vi "Ctor.vi"(8 "error in (no error)":errorcluster, 11 "SinglePlotPanel (type)":refnum<class "RocketPlotPanel.lvclass">) -> (0 "error out":errorcluster, 3 "SinglePlotPanel (running type)":refnum<class "RocketPlotPanel.lvclass">)   [LabVIEW 2021, in "RocketPlot.lvlib" / "RocketPlotPanel.lvclass"]
uses:
  RocketPlotPanel.lvclass
  RocketPlotPanel.lvclass/RocketPlotPanel.ctl
  <vilib>/IlluminatedG/IG OOPanel/OOPanel/Panel/Panel.lvclass
  RocketPlotHandle/RocketPlotHandle.lvclass
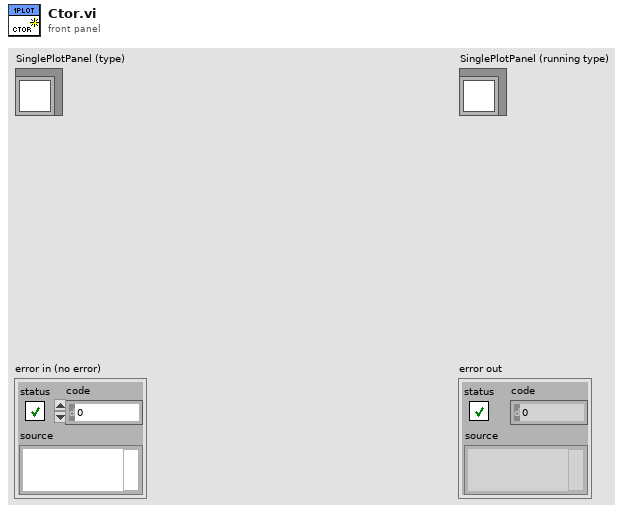
[diagram p1: front panel]
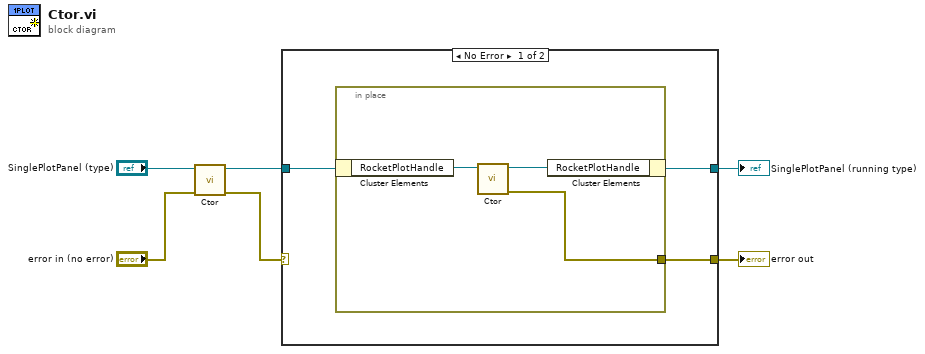
[diagram p0: block diagram]
diagram:
  n1 = call-parent "Ctor.vi"("error in (no error)"="error in (no error)", "Panel in"="SinglePlotPanel (type)") -> ("error out"=w1:errorcluster, "Panel out"=w3:refnum<class "RocketPlotPanel.lvclass">)  [unwired: 8 in]
  n2 = case shown="No Error" w1 {
    selector: w1 -> [_ w14]
    tunnel: [w7 w14] -> w6
    tunnel: [w8 w13] -> w5
    tunnel: w3 -> [w9 w13]
    frame No Error {
      n3 = in-place {
        in-place-border: [w10] -> w7
        n4 = in-place-cluster #1(w9) -> ("RocketPlotHandle"=w12:refnum<class "RocketPlotHandle.lvclass">)
        n5 = call-dynamic "Ctor.vi"("BluePlotHandle in"=w12) -> ("error out"=w10:errorcluster, "BluePlotHandle out"=w11:refnum<class "RocketPlotHandle.lvclass">)  [unwired: 9 in]
        n6 = in-place-cluster #1("RocketPlotHandle"=w11) -> (w8:refnum<class "RocketPlotPanel.lvclass">)
      }
    }
    frame Error {
    }
  }
  "error out" <- w6
  "SinglePlotPanel (running type)" <- w5
